vi "Initialize.vi"(8 "error in (no error)":errorcluster, 10 "Device":string) -> (0 "error out":errorcluster, 3 "DMM out":refnum<class "DMM.lvclass">)   [LabVIEW 2018, in "DMM.lvlib" / "DMM.lvclass"]
uses:
  DMM.lvclass
  DMM.lvclass/DMM.ctl
  PPLs/Configuration/Configuration.lvlibp/Configuration.lvclass
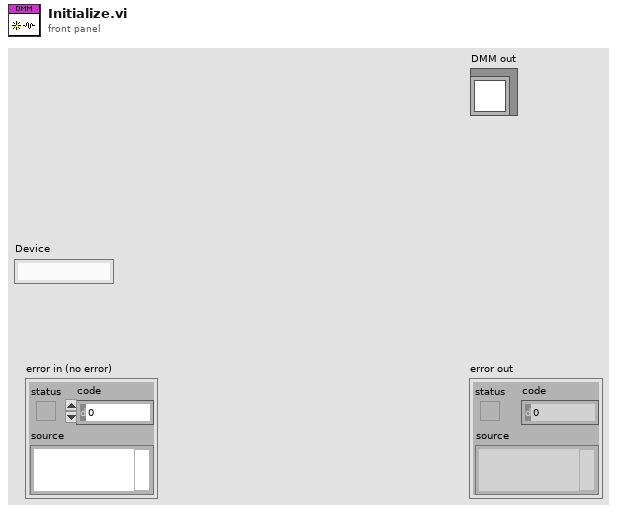
[diagram p1: front panel]
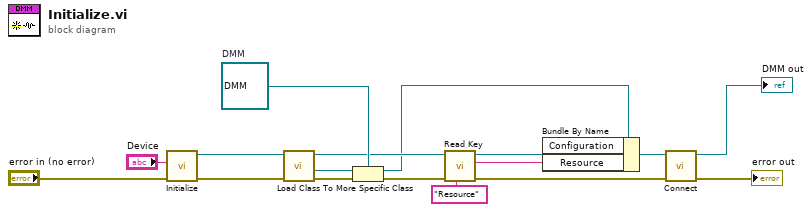
[diagram p0: block diagram]
diagram:
  w10 = refnum<class "DMM.lvclass"> refnum  # DMM
  n1 = call "Initialize.vi"("error in"="error in (no error)", "Device"="Device") -> ("error out"=w14:errorcluster, "Configuration out"=w13:refnum<class "Configuration.lvclass">)  [unwired: 8 in]
  n2 = call "Load Class.vi"("error in"=w14, "Configuration in"=w13) -> ("error out"=w12:errorcluster, "Class out"=w11:refnum<class>, "Configuration out"=w9:refnum<class "Configuration.lvclass">)  [unwired: 7 in]
  n3 = To More Specific Class(target class=w10, reference=w11, error in=w12) -> (specific class reference=w6:refnum<class "DMM.lvclass">, error out=w7:errorcluster)
  n4 = call "Read Key.vi"("Key:"="Resource", "error in"=w7, "Configuration in"=w9) -> ("error out"=w3:errorcluster, "Value"=w4:string, "Configuration out"=w5:refnum<class "Configuration.lvclass">)  [unwired: 6 in]
  n5 = Bundle By Name(cluster=w6, "Configuration"=w5, "Resource"=w4) -> (w2:refnum<class "DMM.lvclass">)
  n6 = call-dynamic "Connect.vi"("error in (no error)"=w3, "DMM in"=w2) -> ("error out"=→"error out":errorcluster, "DMM out"=→"DMM out":refnum<class "DMM.lvclass">)  [unwired: 8 in]
